vi "velocitymode_rev2.vi"() -> ()   [LabVIEW 2018]
uses:
  <vilib>/Platform/TimedLoop/XDataNode/timing_clust.ctl
  <vilib>/Platform/TimedLoop/XDataNode/nitl_modes.ctl
  <vilib>/Platform/TimedLoop/XDataNode/wakeup.ctl
  <vilib>/FPGAPlugInAG/myRIO-1900/niLvFpga_Open_myRIO-1900.vi
  <vilib>/rvi/interface/common/dynamic/niFpgaDynamicAddResources.vi
  <vilib>/FPGAPlugInAG/Dynamic/niLvFpga_Close_Dynamic.vi
  <vilib>/rvi/interface/nirviOpenFPGA/nirviOpenFPGA.xnode
  FPGA Bitfiles/WattBalanceRev1_FPGATarget_FPGASPI2_21rs6YSGst0.lvbitx
  FPGA files/FPGA_SPI.vi
  <vilib>/Platform/TimedLoop/XDataNode/XDataNode.xnode
  <vilib>/rvi/interface/nirviCloseFPGA/nirviCloseFPGA.xnode
  <vilib>/Platform/TimedLoop/XDataNode/XDNodeRunTimeDep.lvlib
panel:
  in  "CH1  2":bool[](array[boolean])=[FALSE, FALSE, TRUE, FALSE, FALSE, TRUE, FALSE, FALSE, FALSE, FALSE, FALSE, FALSE, FALSE, FALSE, FALSE, FALSE]
  in  "CH2 2":bool[](array[boolean])=[FALSE, FALSE, FALSE, FALSE, FALSE, TRUE, FALSE, FALSE, FALSE, FALSE, FALSE, FALSE, FALSE, FALSE, FALSE, FALSE]
  out "Finished Late? [i-1]":bool
  out "BL":dbl(graph)=719.9999999997312
  out "velocity":dbl(graph)=7.629278117707349e-06
  out "prev pos":dbl=-0.00011563849428567067
  in  "delay (us)":i64=500
  in  "no. moving avg.":i32=5
  out "avg loop rate":dbl=1.9807573891625616
  in  "Stop Button":bool
  in  "offset (mV)":dbl=1000.0
  in  "amplitude (V)":dbl
  in  "frequency (Hz)":dbl=0.5
  in  "emf on/off":bool=TRUE
  in  "pos on/off":bool=TRUE
  out "EMF":dbl(graph)=0.005493080244747241
  out "Displacement (m)":dbl(graph)=-4.626089079451301
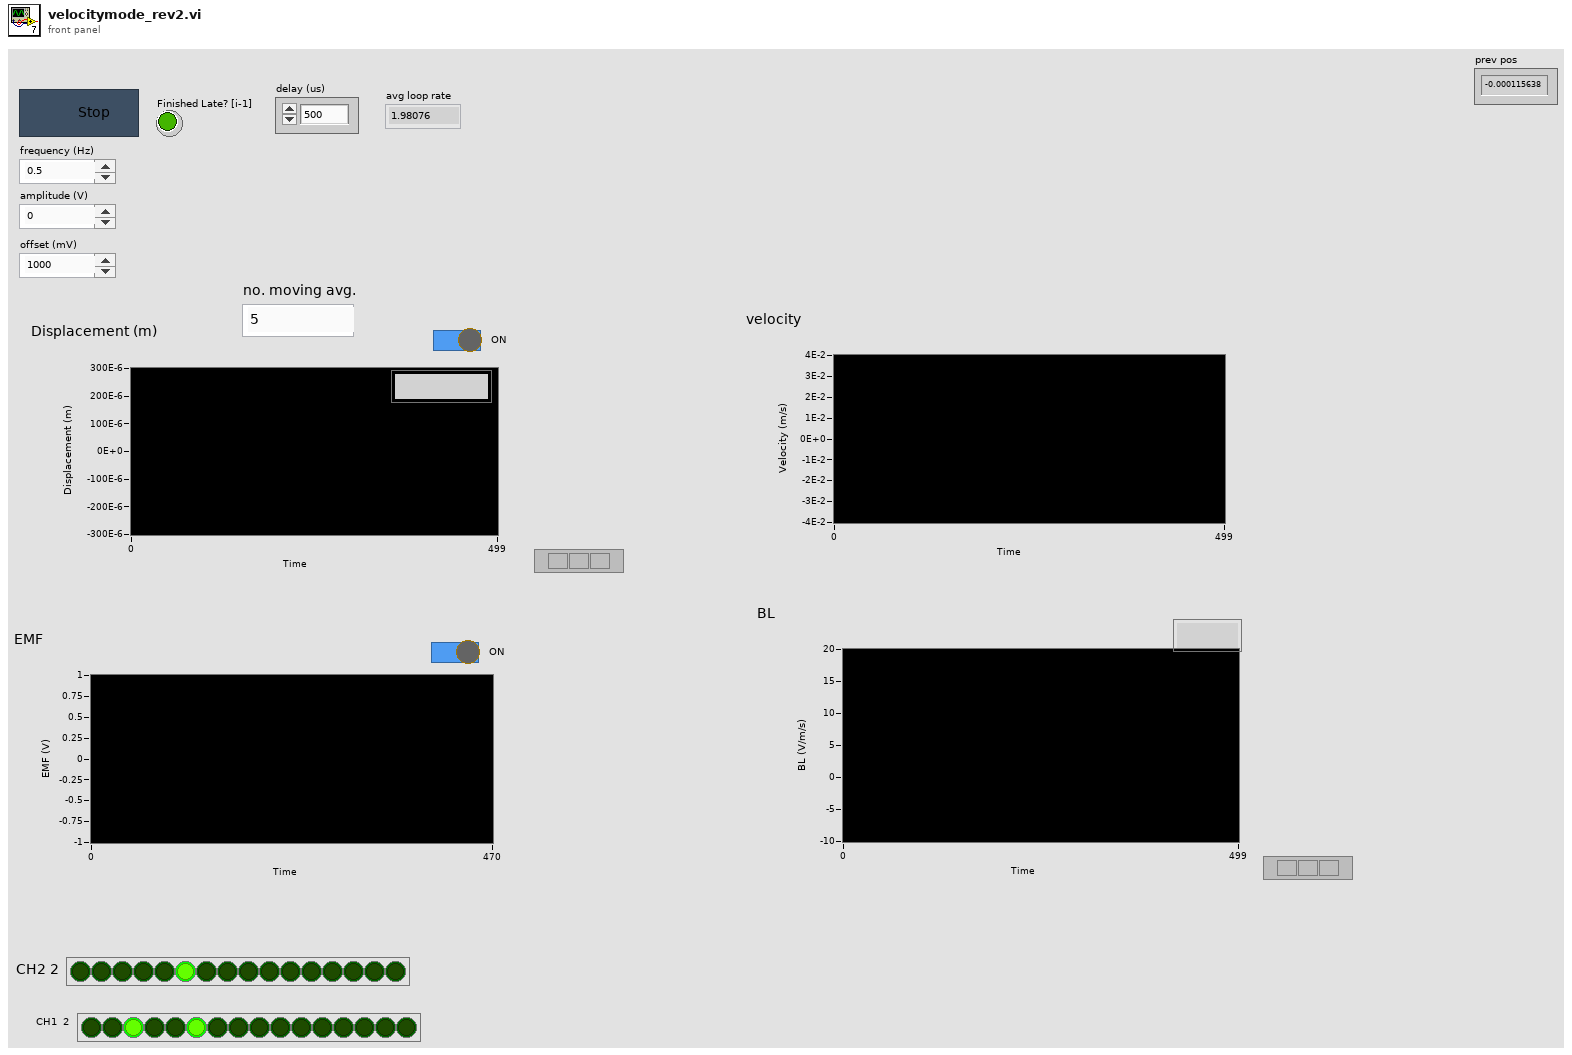
[diagram p1: front panel]
types:
  T1 = typedef "XDNodeRunTimeDep.lvlib/timing_clust.ctl" = cluster{"Expected End [f-1]":u64, "Actual End [f-1]":u64, "Finished Late? [f-1]":bool, "Expected End [i-1]":u64, "Actual End [i-1]":u64, "Finished Late? [i-1]":bool, "Expected Start [i]":u64, "Actual Start [i]":u64, "Expected Start [f]":u64, "Actual Start [f]":u64, "Source Name":string, "Structure Name":string, "Period":i64, "Deadline":i64, "Offset":i64, "Start":i64, "Priority":i32, "Timeout":i32, "Mode":T2, "Wakeup Reason":T3, "Error":errorcluster, "Source Type":string, "Secondary Source Type":string, "Global End Time":u64, "Global Start Time":u64, "Frame Duration":u64, "Iteration Duration":u64, "Assigned CPU":i32, "I/O Scan Engine Mode":u32}
  T2 = typedef "XDNodeRunTimeDep.lvlib/nitl_modes.ctl" = enum32{"No Change", "Process missed periods, maintain original phase", "Discard missed periods, maintain original phase", "Process missed periods, ignore original phase", "Discard missed periods, ignore original phase"}
  T3 = typedef "XDNodeRunTimeDep.lvlib/wakeup.ctl" = enum32{"Normal", "Aborted", "Asynchronous wakeup", "Timing source error", "Timed loop error", "Timeout"}
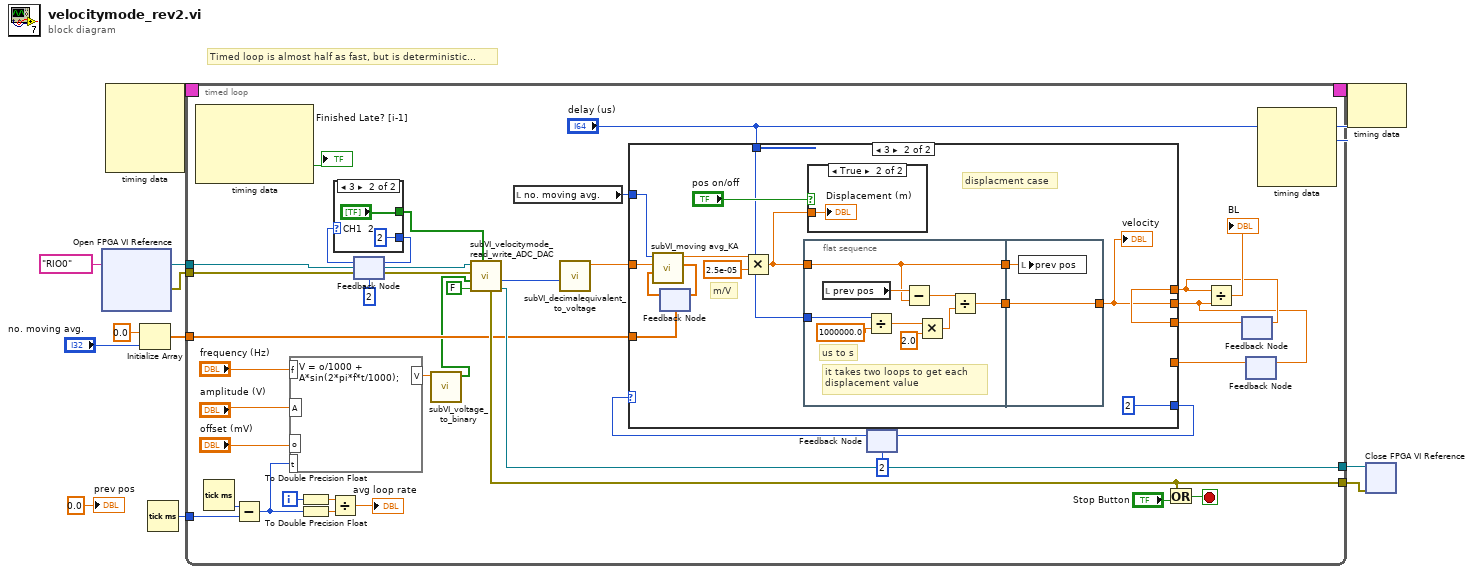
[diagram p0: block diagram]
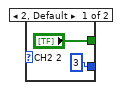
[diagram p2: hidden frame]
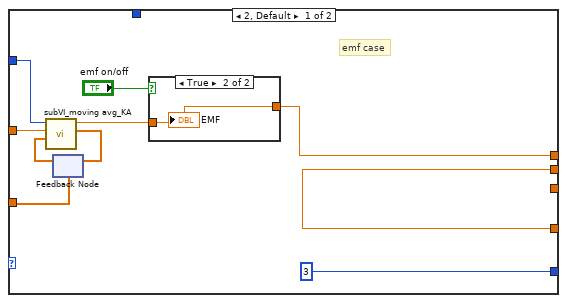
[diagram p3: hidden frame]
diagram:
  # "Timed loop is almost half as fast, but is deterministic..."
  n1 = xnode "Open FPGA VI Reference"("resource name"=tag "RIO0") -> ("FPGA VI Reference Out"=w12:refnum<k20>, "error out"=w11:errorcluster)  [unwired: 1 in]
  n2 = node-c288() -> (w3:T1)  [unwired: 4 in]
  n3 = Initialize Array(0.0 ("element"), "no. moving avg.") -> (w6:dbl[])
  n4 = Tick Count (ms)() -> (millisecond timer value=w4:u32)
  n5 = timed-loop {
    tunnel: w4 -> [w48]
    tunnel: w12 -> [w19]
    tunnel: w11 -> [w40]
    tunnel: [w35] -> w10
    tunnel: [w34] -> w9
    tunnel: w6 -> [w28]
    timing: w3 -> [_]
    timing-out: [_] -> w2
    i -> [w47]
    stop <- w37 stop-if-true
    n6 = node-c288() -> (→"Finished Late? [i-1]":bool)  [unwired: 1 in, 3 out]
    n7 = Tick Count (ms)() -> (millisecond timer value=w49:u32)
    n8 = Subtract(x=w49, y=w48) -> (x-y=w27:u32)
    n9 = formula code="V = o/1000 + \nA*sin(2*pi*f*t/1000);"("f"="frequency (Hz)", "A"="amplitude (V)", "t"=w27, "o"="offset (mV)") -> ("V"=w39:dbl)
    n10 = To Double Precision Float(number=w47) -> (double precision float=w45:dbl)
    n11 = To Double Precision Float(number=w27) -> (double precision float=w46:dbl)
    n12 = Divide(x=w45, y=w46) -> (x/y=→"avg loop rate":dbl)
    n13 = feedback #1(2) -> (w16:i32)
    n14 = case shown="3" w16 {
      tunnel: ["CH2 2" "CH1  2"] -> w15
      tunnel: [3 2] -> w14
      frame 2, Default {
      }
      frame 3 {
      }
    }
    n15 = feedback-in #1(w14) -> ()
    n16 = call "subVI_voltage_to_binary.vi"("voltage"=w39) -> ("binary"=w13:bool[])  [unwired: 10 in]
    n17 = call "subVI_velocitymode_read_write_ADC_DAC.vi"("ADC write"=w15, "read only"=FALSE, "DAC"=w13, "error in"=w40, "FPGA VI Reference In"=w19) -> ("FPGA VI Reference Out"=w35:refnum<k20>, "dec"=w38:u32, "error out"=w34:errorcluster)  [unwired: 2 in, 2 out]
    n18 = local read "no. moving avg."() -> (w30:i32)
    n19 = call "subVI_decimalequivalent_to_voltage.vi"("dec"=w38) -> ("V"=w29:dbl)  [unwired: 10 in]
    n20 = feedback #2(2) -> (w32:i32)
    n21 = Or(x=w34, y="Stop Button") -> (x .or. y?=w37:bool)
    n22 = feedback #3() -> (w25:dbl)  [unwired: 1 in]
    n23 = feedback #4() -> (w24:dbl)  [unwired: 1 in]
    n24 = case shown="3" w32 {
      tunnel: [3 2] -> w33
      tunnel: w30 -> [w64 w83]
      tunnel: w29 -> [w62 w72]
      tunnel: w28 -> [w63 w82]
      tunnel: "delay (us)" -> [_ w78]
      tunnel: [w60 w76] -> w22
      tunnel: [w59 w73] -> w21
      tunnel: w25 -> [_ w76]
      tunnel: w24 -> [w59 _]
      frame 2, Default {
        # "emf case"
        n25 = feedback #5(w63) -> (w67:dbl[])
        n26 = call "subVI_moving avg_KA.vi"("input array"=w67, "sample"=w62, "no. moving avg."=w64) -> ("output array"=w66:dbl[], "avg."=w65:dbl)  [unwired: 7 in]
        n27 = feedback-in #5(w66) -> ()
        n28 = case shown="True" "emf on/off" {
          tunnel: w65 -> [_ w69]
          tunnel: [_ w69] -> w60
          frame False {
          }
          frame True {
            "EMF" <- w69
          }
        }
      }
      frame 3 {
        # "displacment case"
        # "m/V"
        n29 = feedback #6(w82) -> (w80:dbl[])
        n30 = call "subVI_moving avg_KA.vi"("input array"=w80, "sample"=w72, "no. moving avg."=w83) -> ("output array"=w81:dbl[], "avg."=w71:dbl)  [unwired: 7 in]
        n31 = feedback-in #6(w81) -> ()
        n32 = Multiply(x=w71, y=2.5e-05) -> (x*y=w70:dbl)
        n33 = flat-sequence {
          tunnel: w78 -> [w86]
          tunnel: w70 -> [w91]
          tunnel: [w91] -> w77
          tunnel: [w85] -> w74
          tunnel: w77 -> [w95]
          tunnel: w74 -> [w94]
          tunnel: [w94] -> w73
          frame #0 {
            # "us to s"
            # "it takes two loops to get each displacement value"
            n34 = local read "prev pos"() -> (w92:dbl)
            n35 = Divide(x=w86, y=1000000.0) -> (x/y=w88:dbl)
            n36 = Subtract(x=w92, y=w91) -> (x-y=w93:dbl)
            n37 = Multiply(x=w88, y=2.0 ("x")) -> (x*y=w87:dbl)
            n38 = Divide(x=w93, y=w87) -> (x/y=w85:dbl)
          }
          frame #1 {
            n39 = local write "prev pos"(w95) -> ()
          }
        }
        n40 = case shown="True" "pos on/off" {
          tunnel: w70 -> [_ w96]
          frame False {
          }
          frame True {
            "Displacement (m)" <- w96
          }
        }
        "velocity" <- w73
      }
    }
    n41 = feedback-in #2(w33) -> ()
    n42 = Divide(x=w22, y=w21) -> (x/y=→"BL":dbl)
    n43 = feedback-in #3(w22) -> ()
    n44 = feedback-in #4(w21) -> ()
    n45 = node-c288("delay (us)") -> ()  [unwired: 3 in, 1 out]
  }
  n46 = node-c288(w2) -> ()  [unwired: 1 out]
  n47 = xnode "Close FPGA VI Reference"("FPGA VI Reference In"=w10, "error in"=w9) -> ()  [unwired: 1 out]
  "prev pos" <- 0.0
